vi "73_Vision_RC Servo_DC_Moto_1.vi"() -> ()   [LabVIEW 2018]
uses:
  <userlib>/KNR OS 4.0 LabVIEW Toolkit/Type Definition/Resource.ctl
  <userlib>/KNR OS 4.0 LabVIEW Toolkit/Type Definition/RC Servo Port.ctl
  <userlib>/KNR OS 4.0 LabVIEW Toolkit/Type Definition/DC Motor Port.ctl
panel:
  out "area":dbl
  out "RC Pulse Width (uS)":u16[](array[numeric])
  out "Image Out":T1(plugin-control)
  in  "stop":bool
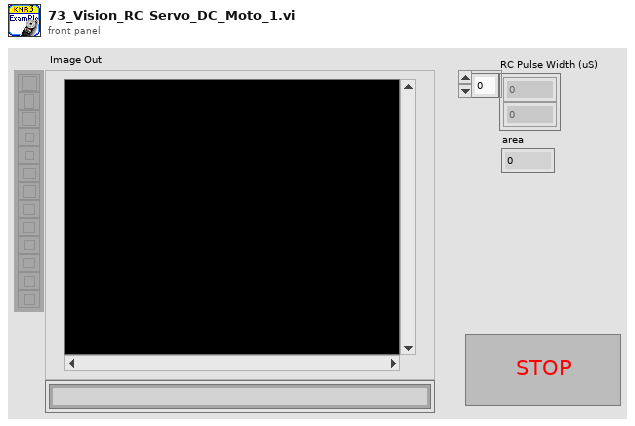
[diagram p1: front panel]
types:
  T1 = typedef "IMAQ Image.ctl" = refnum<image>
  T2 = typedef "RC Servo Port.ctl" = u16
  T3 = typedef "Resource.ctl" = enum16{"KNRm_DDRC", "KNRm_DDDD", "KNRm_DDDR", "KNRm_DDDC", "KNR", "KNRm_neww"}
  T4 = typedef "KNR3 Reference.ctl" = cluster{"FPGA Session":refnum<class "FPGA Interface Base.lvclass">, "Resource":T3}
  T5 = typedef "DC Motor Port.ctl" = u16
  T6 = cluster{"Left":dbl, "Top":dbl, "Right":dbl, "Bottom":dbl}
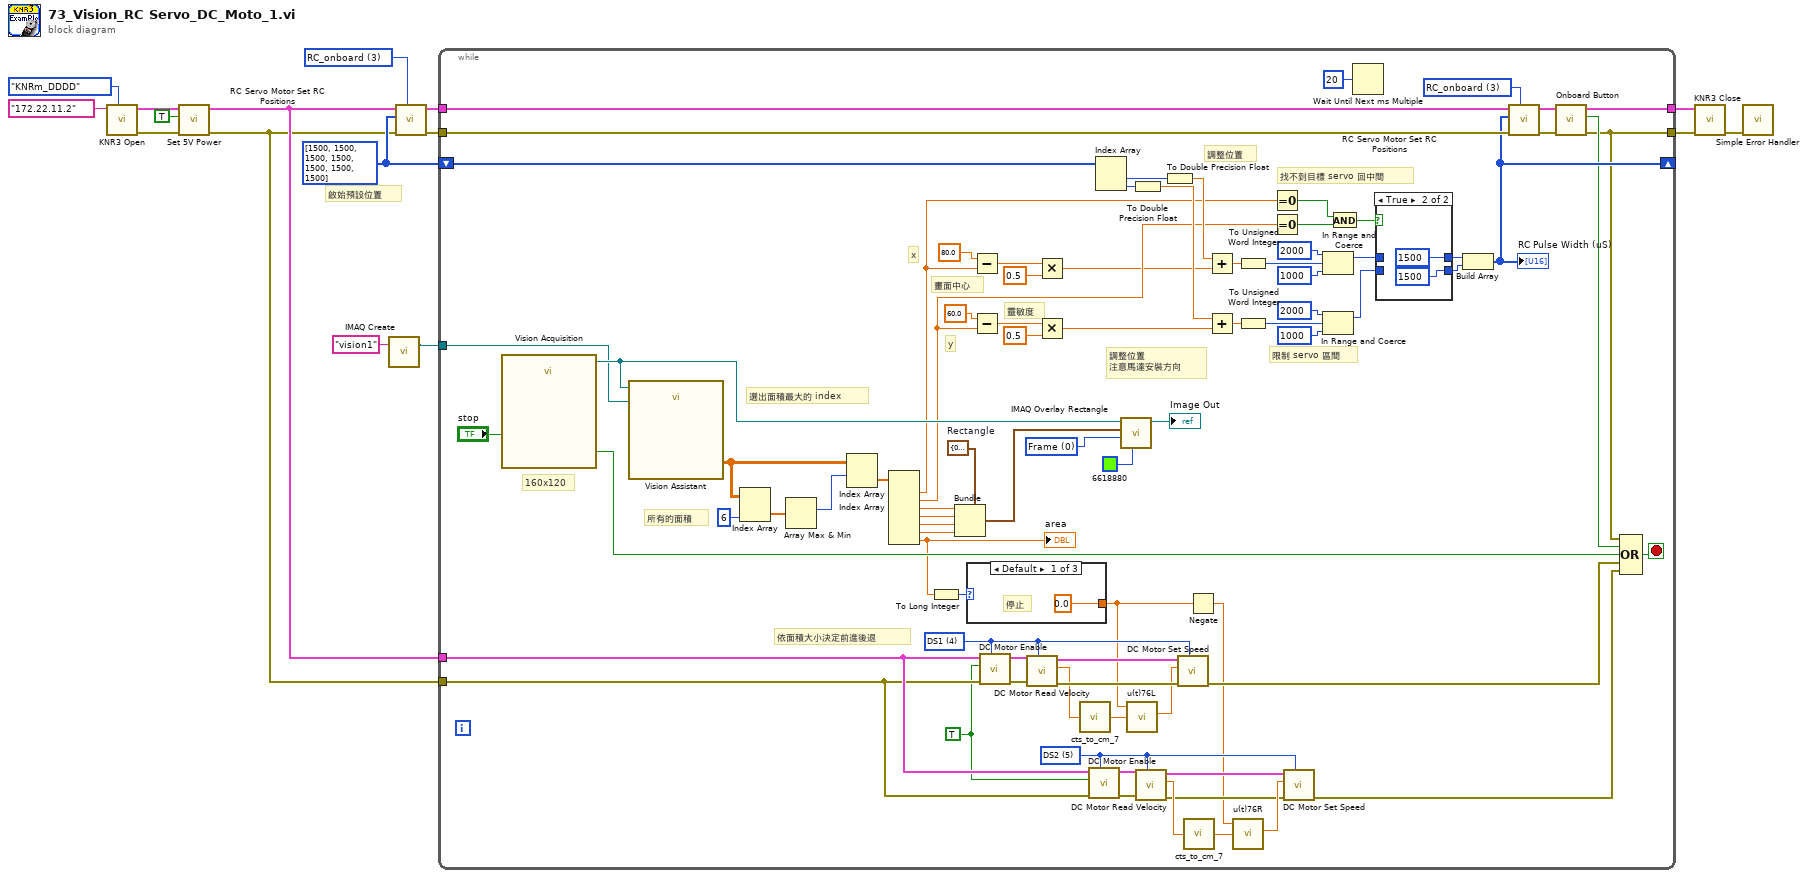
[diagram p0: block diagram]
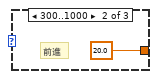
[diagram p2: hidden frame]
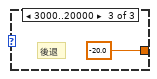
[diagram p3: hidden frame]
diagram:
  w3 = u16[] [1500, 1500, 1500, 1500, 1500, 1500, 1500] ("RC Pulse Width (1500 uS)")
  w6 = T2 3 items=["RC_onboard"=3, "RC_box"=9] ("Port (RC_onboard)")
  # "啟始預設位置"
  n1 = call <userlib>:"KNR3 Open.vi"("Resource"=Resource."KNRm_DDDD", "IP"="172.22.11.2") -> ("error out"=w14:errorcluster, "KNR out"=w15:T4)  [unwired: 8 in]
  n2 = call <userlib>:"Set 5V Power.vi"("error in (no error)"=w14, "5V Power(T)"=TRUE ("5V Power"), "KNR in"=w15) -> ("error out"=w1:errorcluster, "KNR out"=w2:T4)  [unwired: 7 in]
  n3 = call "IMAQ Create"("Image Name"="vision1") -> ("New Image"=w4:T1)  [unwired: 4 in, 1 out]
  n4 = call <userlib>:"RC Servo Motor Set RC Positions.vi"("Port (RC_onboard)"=w6, "RC Pulse Width (1500 uS)"=w3, "KNR in"=w2) -> ("KNR out"=w7:T4)  [unwired: 7 in, 1 out]
  n5 = while {
    tunnel: w7 -> [w98]
    tunnel: [w19] -> w9
    tunnel: w1 -> [w96]
    tunnel: [w17] -> w8
    tunnel: w4 -> [w78]
    shift-right: [w62] -> _
    shift-left: w3 -> [w65]
    tunnel: w2 -> [w26]
    tunnel: w1 -> [w25]
    stop <- w95 stop-if-true
    w23 = u32 0 items=["Frame", "Fill", "Highlight"] ("Drawing Mode (Frame)")
    w29 = T5 5 items=["DS1"=4, "DS2"=5, "DS3"=6, "DS4"=7] ("Port 2")
    w20 = TRUE ("Enable Motor(F)")
    w44 = T5 4 items=["DS1"=4, "DS2"=5, "DS3"=6, "DS4"=7] ("Port 2")
    w91 = T6 {"Left"=0.0, "Top"=0.0, "Right"=0.0, "Bottom"=0.0}  # Rectangle
    w93 = T2 3 items=["RC_onboard"=3, "RC_box"=9] ("RC Motor")
    # "調整位置\n注意馬達安裝方向"
    # "依面積大小決定前進後退"
    # "調整位置"
    # "靈敏度"
    # "所有的面積"
    # "畫面中心"
    # "限制 servo 區間"
    # "找不到目標 servo 回中間"
    # "y"
    # "x"
    # "160x120"
    # "選出面積最大的 index"
    n6 = call "Vision Acquisition"("Stop (F)"="stop") -> ("Image Out"=w83:T1, "Stopped"=w76:bool)  [unwired: 24 in, 1 out]
    n7 = call "Vision Assistant"("Image In"=w83, "Image Dst"=w78) -> ("Particle Measurements (Pixels) (Particle Analysis 1)"=w82:dbl[][])  [unwired: 22 in, 3 out]
    n8 = Index Array "Index Array"(array=w82, index (col)=6 ("disabled index (col)")) -> (element=w81:dbl[])  [unwired: 1 in]
    n9 = Array Max & Min(array=w81) -> (max index (indices)=w80:i32)  [unwired: 3 out]
    n10 = Index Array "Index Array"(array=w82, index (row)=w80) -> (element=w92:dbl[])  [unwired: 1 in]
    n11 = Index Array "Index Array"(array=w92) -> (element #1=w55:dbl, element #2=w54:dbl, element #3=w90:dbl, element #4=w89:dbl, element #5=w88:dbl, element #6=w87:dbl, element #7=w37:dbl)  [unwired: 7 in]
    "area" <- w37
    n12 = To Long Integer(number=w37) -> (32bit integer=w22:i32)
    n13 = Bundle "Bundle"(cluster=w91, "Left"=w90, "Top"=w89, "Right"=w88, "Bottom"=w87) -> (w86:T6)
    n14 = case shown="Default" w22 {
      tunnel: [0.0 20.0 -20.0] -> w16
      frame Default {
        # "停止"
      }
      frame 300..1000 {
        # "前進"
      }
      frame 3000..20000 {
        # "後退"
      }
    }
    n15 = Subtract(x=80.0 ("y"), y=w55) -> (x-y=w72:dbl)
    n16 = Subtract(x=60.0 ("y"), y=w54) -> (x-y=w73:dbl)
    n17 = call <userlib>:"DC Motor Enable.vi"("Port (DS1)"=w44, "error in (no error)"=w25, "Enable Motor(F)"=w20, "KNR in"=w26) -> ("error out"=w40:errorcluster, "KNR out"=w39:T4)  [unwired: 6 in]
    n18 = call <userlib>:"DC Motor Read Velocity.vi"("Port (DS1)"=w44, "error in (no error)"=w40, "KNR in"=w39) -> ("error out"=w43:errorcluster, "Velocity (cts/sec)"=w41:dbl, "KNR out"=w42:T4)  [unwired: 6 in]
    n19 = Multiply(x=w72, y=0.5) -> (x*y=w53:dbl)
    n20 = Multiply(x=w73, y=0.5) -> (x*y=w52:dbl)
    n21 = call "cts_to_cm_7.vi"("cts"=w41) -> ("cm"=w21:dbl)
    n22 = call <userlib>:"DC Motor Enable.vi"("Port (DS1)"=w29, "error in (no error)"=w25, "Enable Motor(F)"=w20, "KNR in"=w26) -> ("error out"=w33:errorcluster, "KNR out"=w34:T4)  [unwired: 6 in]
    n23 = Index Array "Index Array"(array=w65) -> (element #1=w64:u16, element #2=w63:u16)  [unwired: 2 in]
    n24 = call "IMAQ Overlay Rectangle"("Color"=u32 6618880, "Drawing Mode (Frame)"=w23, "Rectangle"=w86, "Image"=w83) -> ("Image Out"=→"Image Out":T1)  [unwired: 6 in, 1 out]
    n25 = call "u(t)76L.vi"("Velocity"=w21, "Desire Velosity"=w16) -> ("u(t)"=w38:dbl)  [unwired: 6 in]
    n26 = To Double Precision Float(number=w63) -> (double precision float=w56:dbl)
    n27 = call <userlib>:"DC Motor Read Velocity.vi"("Port (DS1)"=w29, "error in (no error)"=w33, "KNR in"=w34) -> ("error out"=w30:errorcluster, "Velocity (cts/sec)"=w32:dbl, "KNR out"=w31:T4)  [unwired: 6 in]
    n28 = To Double Precision Float(number=w64) -> (double precision float=w57:dbl)
    n29 = call <userlib>:"DC Motor Set Speed.vi"("Port (DS1)"=w44, "error in (no error)"=w43, "Speed (+-100%)"=w38, "KNR in"=w42) -> ("error out"=w28:errorcluster)  [unwired: 6 in, 1 out]
    n30 = call "cts_to_cm_7.vi"("cts"=w32) -> ("cm"=w36:dbl)
    n31 = Negate(x=w16) -> (-x=w24:dbl)
    n32 = Add(x=w57, y=w53) -> (x+y=w74:dbl)
    n33 = Add(x=w56, y=w52) -> (x+y=w75:dbl)
    n34 = call "u(t)76R.vi"("Desire Velosity"=w24, "Velocity"=w36) -> ("u(t)"=w35:dbl)  [unwired: 5 in]
    n35 = To Unsigned Word Integer(number=w74) -> (unsigned 16bit integer=w59:u16)
    n36 = To Unsigned Word Integer(number=w75) -> (unsigned 16bit integer=w58:u16)
    n37 = Equal To 0?(x=w55) -> (x = 0?=w49:bool)
    n38 = Equal To 0?(x=w54) -> (x = 0?=w50:bool)
    n39 = call <userlib>:"DC Motor Set Speed.vi"("Port (DS1)"=w29, "error in (no error)"=w30, "Speed (+-100%)"=w35, "KNR in"=w31) -> ("error out"=w27:errorcluster)  [unwired: 6 in, 1 out]
    n40 = In Range and Coerce(upper limit=u16 2000, x=w59, lower limit=u16 1000) -> (coerced(x)=w48:u16)  [unwired: 1 out]
    n41 = In Range and Coerce(upper limit=u16 2000, x=w58, lower limit=u16 1000) -> (coerced(x)=w47:u16)  [unwired: 1 out]
    n42 = And(x=w49, y=w50) -> (x .and. y?=w51:bool)
    n43 = Wait Until Next ms Multiple(millisecond multiple=u32 20) -> ()  [unwired: 1 out]
    n44 = case shown="True" w51 {
      tunnel: w48 -> [w103 _]
      tunnel: w47 -> [w102 _]
      tunnel: [w103 u16 1500] -> w46
      tunnel: [w102 u16 1500] -> w45
      frame False {
      }
      frame True {
      }
    }
    n45 = Build Array "Build Array"(w46, w45) -> (w62:u16[])
    "RC Pulse Width (uS)" <- w62
    n46 = call <userlib>:"RC Servo Motor Set RC Positions.vi"("Port (RC_onboard)"=w93, "error in (no error)"=w96, "RC Pulse Width (1500 uS)"=w62, "KNR in"=w98) -> ("error out"=w17:errorcluster, "KNR out"=w97:T4)  [unwired: 6 in]
    n47 = call <userlib>:"Onboard Button.vi"("KNR in"=w97) -> ("value"=w18:bool, "KNR out"=w19:T4)  [unwired: 8 in, 1 out]
    n48 = Compound Arithmetic op=OR(w17, w18, w76, w28, w27) -> (w95:bool)
  }
  n49 = call <userlib>:"KNR3 Close.vi"("error in (no error)"=w8, "KNR in"=w9) -> ("error out"=w13:errorcluster)  [unwired: 9 in]
  n50 = call <vilib>:"Simple Error Handler.vi"("error in (no error)"=w13) -> ()  [unwired: 4 in, 5 out]
